vi "ResizeTabControltoPane.vi"(4 "Force aspect ratio?":bool, 5 "Borders in Percent(T) or Pixels (F)":bool, 6 "Adjust":u16(ring) items=["Height", "Width", "Both"], 7 "Minimal":T1, 8 "error in (no error)":errorcluster, 9 "Borders":T2, 10 "TabControl":refnum<vi>, 11 "PentaPanesGUI in":refnum<class "PentaPanes.lvclass">) -> (0 "error out":errorcluster, 3 "PentaPanesGUI out":refnum<class "PentaPanes.lvclass">)   [LabVIEW 2022 SP3, in "PentaPanesLibrary.lvlib" / "PentaPanes.lvclass"]
uses:
  PentaPanes.lvclass
  BordersCluster.ctl
  <vilib>/Utility/miscctls.llb/LVBoundsTypeDef.ctl
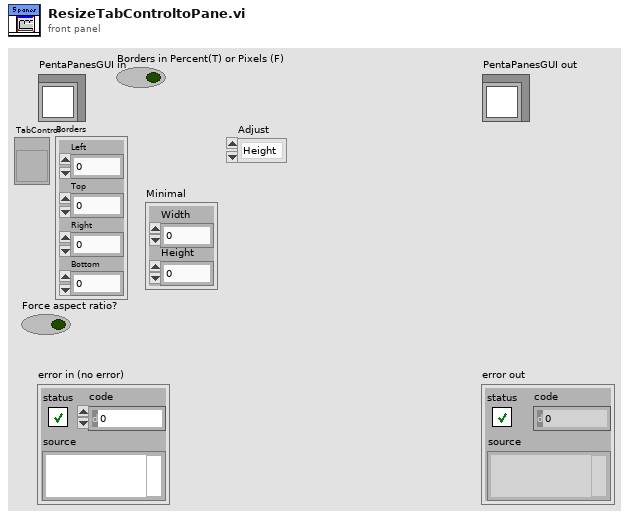
[diagram p1: front panel]
types:
  T1 = typedef "LVBoundsTypeDef.ctl" = cluster{"Width":i32, "Height":i32}
  T2 = typedef "PentaPanesLibrary.lvlib/PentaPanes.lvclass/BordersCluster.ctl" = cluster{"Left":i32, "Top":i32, "Right":i32, "Bottom":i32}
  T3 = typedef "LVBoundsTypeDef.ctl" = cluster{"Width":u32, "Height":u32}
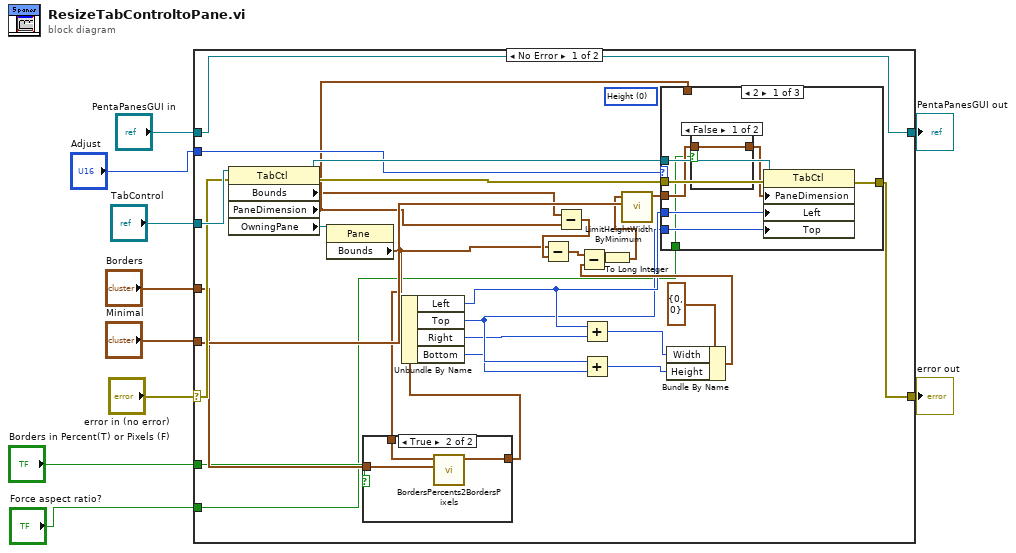
[diagram p0: block diagram]
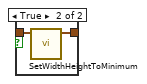
[diagram p3: hidden frame]
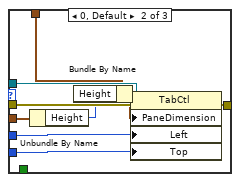
[diagram p4: hidden frame]
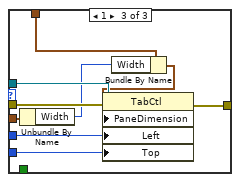
[diagram p5: hidden frame]
diagram:
  n1 = case shown="No Error" "error in (no error)" {
    selector: "error in (no error)" -> [w35 w74]
    tunnel: [w28 w74] -> w9
    tunnel: [w14 w73] -> w7
    tunnel: "PentaPanesGUI in" -> [w14 w73]
    tunnel: "TabControl" -> [w36 _]
    tunnel: "Borders" -> [w19 _]
    tunnel: "Adjust" -> [w27 _]
    tunnel: "Minimal" -> [w25 _]
    tunnel: "Borders in Percent(T) or Pixels (F)" -> [w17 _]
    tunnel: "Force aspect ratio?" -> [w15 _]
    frame No Error {
      (unwired) u16 0 items=["Height", "Width", "Both"] ("Adjust")
      n2 = property class="TabCtl"(reference=w36, error in=w35) -> (reference out=w37:refnum<vi>, error out=w29:errorcluster, "Bounds"=w11:T3, "PaneDimension"=w16:T3, "OwningPane"=w38:refnum<vi>)
      n3 = property class="Pane"(reference=w38) -> ("Bounds"=w22:T3)  [unwired: 1 in, 2 out]
      n4 = case shown="True" w17 {
        tunnel: w22 -> [_ w43]
        tunnel: w19 -> [w40 w42]
        tunnel: [w40 w41] -> w18
        frame False {
        }
        frame True {
          n5 = call "BordersPercents2BordersPixels.vi"("Borders in"=w42, "Bounds"=w43) -> ("Borders out"=w41:T2)  [unwired: 9 in]
        }
      }
      n6 = Unbundle By Name(w18) -> ("Left"=w24:i32, "Top"=w23:i32, "Right"=w21:i32, "Bottom"=w20:i32)
      n7 = Subtract(x=w11, y=w16) -> (x-y=w39:T3)
      n8 = Subtract(x=w22, y=w39) -> (x-y=w31:T3)
      n9 = Add(x=w24, y=w21) -> (x+y=w33:i32)
      n10 = Add(x=w23, y=w20) -> (x+y=w32:i32)
      n11 = Bundle By Name(cluster=T1 {"Width"=0, "Height"=0} ("x-y"), "Width"=w33, "Height"=w32) -> (w30:T1)
      n12 = Subtract(x=w31, y=w30) -> (x-y=w13:T3)
      n13 = To Long Integer(number=w13) -> (32bit integer=w12:cluster{"Width":i32, "Height":i32})
      n14 = call "LimitHeightWidthByMinimum.vi"("Minimal"=w25, "Height Width in"=w12) -> ("Limited Height Width out"=w26:T1)  [unwired: 9 in]
      n15 = case shown="2" w27 {
        tunnel: w37 -> [w51 w63 w72]
        tunnel: w26 -> [w46 w58 w67]
        tunnel: w24 -> [w50 w62 w71]
        tunnel: w23 -> [w49 w61 w70]
        tunnel: w29 -> [w48 w60 w69]
        tunnel: [w47 w59 w68] -> w28
        tunnel: w16 -> [_ w56 w66]
        tunnel: w15 -> [w44 _ _]
        frame 2 {
          n16 = case shown="False" w44 {
            tunnel: w46 -> [w52 w54]
            tunnel: [w52 w53] -> w45
            frame False {
            }
            frame True {
              n17 = call "SetWidthHeightToMinimum.vi"("Limited Height Width in"=w54) -> ("Limited Height Width out"=w53:T1)  [unwired: 10 in]
            }
          }
          n18 = property class="TabCtl"(reference=w51, error in=w48, "PaneDimension"=w45, "Left"=w50, "Top"=w49) -> (error out=w47:errorcluster)  [unwired: 1 out]
        }
        frame 0, Default {
          n19 = Unbundle By Name(w58) -> ("Height"=w55:i32)
          n20 = Bundle By Name(cluster=w56, "Height"=w55) -> (w57:T3)
          n21 = property class="TabCtl"(reference=w63, error in=w60, "PaneDimension"=w57, "Left"=w62, "Top"=w61) -> (error out=w59:errorcluster)  [unwired: 1 out]
        }
        frame 1 {
          n22 = Unbundle By Name(w67) -> ("Width"=w65:i32)
          n23 = Bundle By Name(cluster=w66, "Width"=w65) -> (w64:T3)
          n24 = property class="TabCtl"(reference=w72, error in=w69, "PaneDimension"=w64, "Left"=w71, "Top"=w70) -> (error out=w68:errorcluster)  [unwired: 1 out]
        }
      }
    }
    frame Error {
    }
  }
  "error out" <- w9
  "PentaPanesGUI out" <- w7
